vi "Configure Trigger Source.vi"(8 "error in (no error)":errorcluster, 9 "Trigger Type":u16(ring) items=["Edge", "Pulse", "TV", "Pattern"], 10 "Trigger Source (1: Channel 1)":u16(ring)=1 items=["Channel 1"=1, "Channel 2"=2, "Channel 3"=3, "Channel 4"=4, "External"=5, "External 5"=6, "AC Line"=7], 11 "VISA resource name":refnum<visa-resource-name>) -> (0 "error out":errorcluster, 3 "VISA resource name out":refnum<visa-resource-name>)   [LabVIEW 2010, in "Agilent DSO1000 Series.lvlib"]
doc: "This VI configures trigger source."
uses:
  <instrlib>/Agilent DSO1000 Series/Agilent DSO1000 Series.lvlib
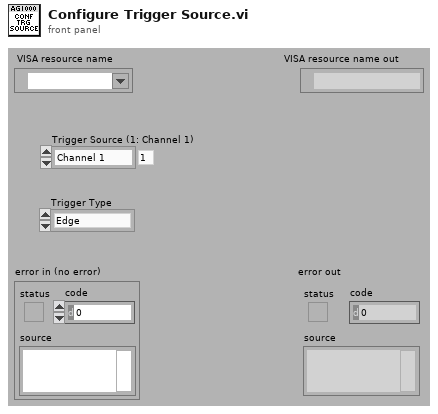
[diagram p1: front panel]
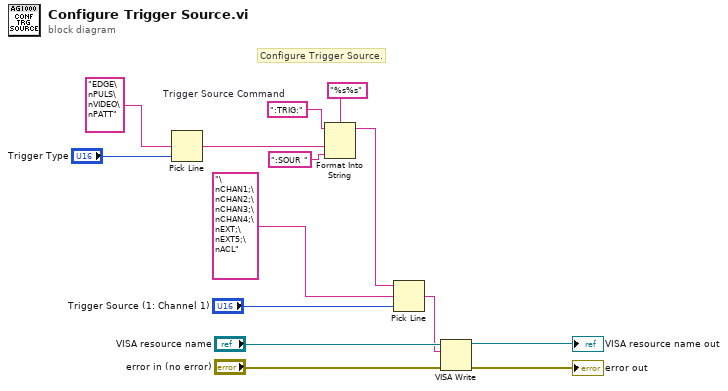
[diagram p0: block diagram]
diagram:
  w7 = ":TRIG:"  # Trigger Source Command
  # "Configure Trigger Source."
  n1 = Pick Line(multi-line string="EDGE\nPULS\nVIDEO\nPATT", line index="Trigger Type") -> (output string=w4:string)  [unwired: 1 in]
  n2 = Format Into String(format string="%s%s", initial string=w7, w4, ":SOUR ") -> (resulting string=w1:string)  [unwired: 1 in, 1 out]
  n3 = Pick Line(string ("")=w1, multi-line string="\nCHAN1;\nCHAN2;\nCHAN3;\nCHAN4;\nEXT;\nEXT5;\nACL", line index="Trigger Source (1: Channel 1)") -> (output string=w10:string)
  n4 = VISA Write(VISA resource name="VISA resource name", write buffer=w10, error in (no error)="error in (no error)") -> (VISA resource name out=→"VISA resource name out":refnum<visa-resource-name>, error out=→"error out":errorcluster)  [unwired: 1 out]
